vi "Manipulator Get Dynamics.vi"(8 "error in (no error)":errorcluster, 11 "VISA resource in":refnum<visa-resource-name>="COM1") -> (0 "error out":errorcluster, 2 "output cluster":cluster{i32, i32, i32}, 3 "VISA resource out":refnum<visa-resource-name>)   [LabVIEW 2012, in "Scientifica Manipulator Daemon.lvlib"]
uses:
  Scientifica Manipulator Daemon.lvlib
panel:
  in  "Dummy Cluster":T1
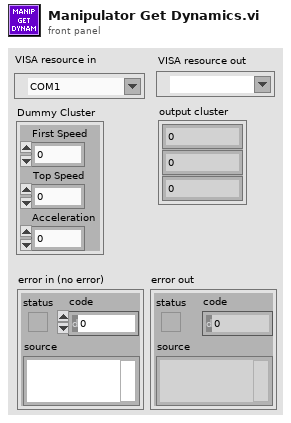
[diagram p1: front panel]
types:
  T1 = cluster{"First Speed":i32, "Top Speed":i32, "Acceleration":i32}
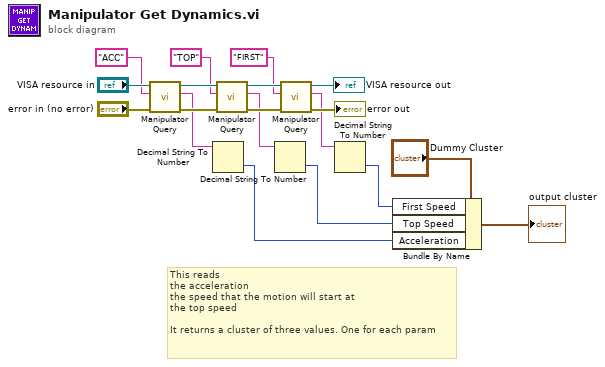
[diagram p0: block diagram]
diagram:
  # "This reads \nthe acceleration\nthe speed that the motion will start at \nthe top speed\n\nIt returns a cluster of three values. One for each param"
  n1 = call "Manipulator Query.vi"("error in (no error)"="error in (no error)", "Command"="ACC", "VISA resource in"="VISA resource in") -> ("error out"=w16:errorcluster, "Response"=w3:string, "VISA resource out"=w17:refnum<visa-resource-name>)  [unwired: 5 in, 1 out]
  n2 = Decimal String To Number(string=w3) -> (number=w5:i32)  [unwired: 2 in, 1 out]
  n3 = call "Manipulator Query.vi"("error in (no error)"=w16, "Command"="TOP", "VISA resource in"=w17) -> ("error out"=w14:errorcluster, "Response"=w2:string, "VISA resource out"=w15:refnum<visa-resource-name>)  [unwired: 5 in, 1 out]
  n4 = Decimal String To Number(string=w2) -> (number=w6:i32)  [unwired: 2 in, 1 out]
  n5 = call "Manipulator Query.vi"("error in (no error)"=w14, "Command"="FIRST", "VISA resource in"=w15) -> ("error out"=→"error out":errorcluster, "Response"=w1:string, "VISA resource out"=→"VISA resource out":refnum<visa-resource-name>)  [unwired: 5 in, 1 out]
  n6 = Decimal String To Number(string=w1) -> (number=w7:i32)  [unwired: 2 in, 1 out]
  n7 = Bundle By Name(cluster="Dummy Cluster", "First Speed"=w7, "Top Speed"=w6, "Acceleration"=w5) -> (→"output cluster":T1)
